vi "Is Empty.vi"(3 "MsgPackArray in":refnum<class "MsgPackArray.lvclass">) -> (1 "Is empty?":bool=TRUE)   [LabVIEW 2020, in "MessagePack.lvlib" / "MsgPackArray.lvclass"]
uses:
  MsgPackArray.lvclass
  MsgPackArray.lvclass/MsgPackArray.ctl
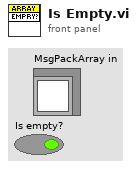
[diagram p1: front panel]
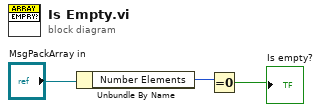
[diagram p0: block diagram]
diagram:
  n1 = Unbundle By Name("MsgPackArray in") -> ("Number Elements"=w2:u32)
  n2 = Equal To 0?(x=w2) -> (x = 0?=→"Is empty?":bool)
